vi "get analog data.vi"(8 "error in (no error)":errorcluster, 10 "analog_data":T1, 11 "id":i32) -> (0 "error out":errorcluster, 2 "analog_data out":T1, 3 "function return":i32)   [LabVIEW 2012, in "libximc.lvlib"]
doc: "result_t XIMC_API get_analog_data (device_t id, analog_data_t* analog_data);"
uses:
  libximc.lvlib
  libximc.dll
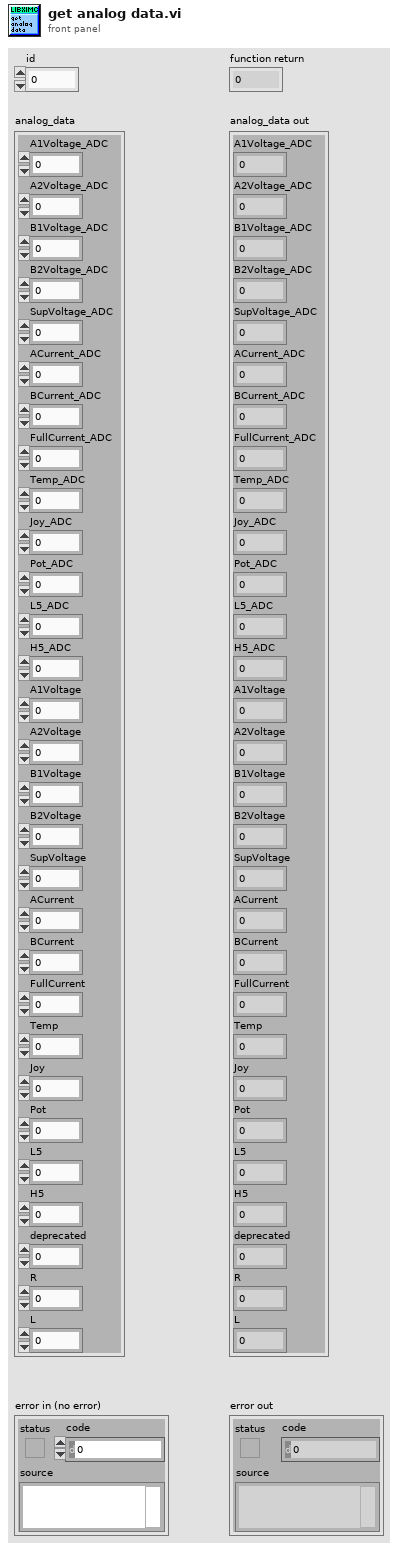
[diagram p1: front panel]
types:
  T1 = cluster{"A1Voltage_ADC":u32, "A2Voltage_ADC":u32, "B1Voltage_ADC":u32, "B2Voltage_ADC":u32, "SupVoltage_ADC":u32, "ACurrent_ADC":u32, "BCurrent_ADC":u32, "FullCurrent_ADC":u32, "Temp_ADC":u32, "Joy_ADC":u32, "Pot_ADC":u32, "L5_ADC":u32, "H5_ADC":u32, "A1Voltage":i32, "A2Voltage":i32, "B1Voltage":i32, "B2Voltage":i32, "SupVoltage":i32, "ACurrent":i32, "BCurrent":i32, "FullCurrent":i32, "Temp":i32, "Joy":i32, "Pot":i32, "L5":i32, "H5":i32, "deprecated":u32, "R":i32, "L":i32}
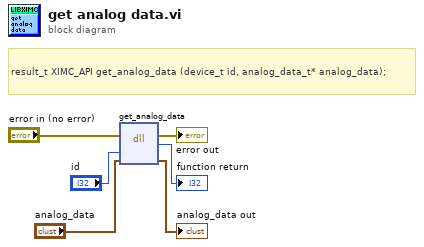
[diagram p0: block diagram]
diagram:
  # "result_t XIMC_API get_analog_data (device_t id, analog_data_t* analog_data);"
  n1 = dll-call lib="C:/Users/Stepan/Downloads/labview_2.9.11_testgen_thread/libximc.*" fn="get_analog_data"(error in="error in (no error)", "id"="id", "analog_data"="analog_data") -> (error out=→"error out":errorcluster, →"function return":i32, "analog_data"=→"analog_data out":T1)  [unwired: 3 in, 1 out]
